vi "dvp Vi Get Packet Size Sel.vi"(10 "pPacketSizeSel":u32, 11 "handle":u32) -> (2 "pPacketSizeSel out":u32, 3 "function return":u32(ring))   [LabVIEW 2018, in "LabViewDVPCamera.lvlib"]
doc: "LabviewDvp2Api dvpStatus dvpViGetPacketSizeSel(dvpHandle handle, dvpUint32 *pPacketSizeSel);"
uses:
  LabViewDVPCamera.lvlib
  LabViewDVPCamera/LabViewDVPCamera.dll
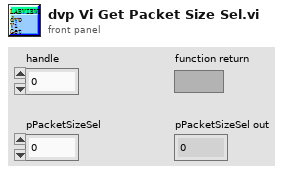
[diagram p1: front panel]
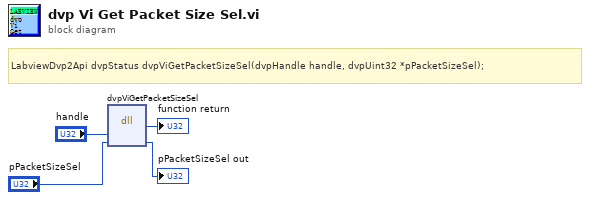
[diagram p0: block diagram]
diagram:
  # "LabviewDvp2Api dvpStatus dvpViGetPacketSizeSel(dvpHandle handle, dvpUint32 *pPacketSizeSel);"
  n1 = dll-call lib="C:/Program Files (x86)/DVP2 Labview cn 64/Sample/LabViewDVPCamera/LabViewDVPCamera.*" fn="dvpViGetPacketSizeSel"("handle"="handle", "pPacketSizeSel"="pPacketSizeSel") -> (→"function return":u32, "pPacketSizeSel"=→"pPacketSizeSel out":u32)  [unwired: 4 in, 2 out]
